vi "Get Field.vi"(0 "Z-Axis Communications Config":T1={"GPIB address"=22, "GPIB bus"=0, "connection ID"=refnum, "IP"="111.111.111.1", "Active Comm Interface"=0, "Serial Port"="", "Programmer Type"=0} {"Active Comm Interface" items=["TCP/IP (Model 430 Only)", "RS232", "IEEE488"]; "Programmer Type" items=["Model 430", "Model 420"]}, 3 "error in":T2) -> (4 "Response":bool, 6 "Field(T)":dbl format="%.3f", 8 "error out":T2)   [LabVIEW 2019]
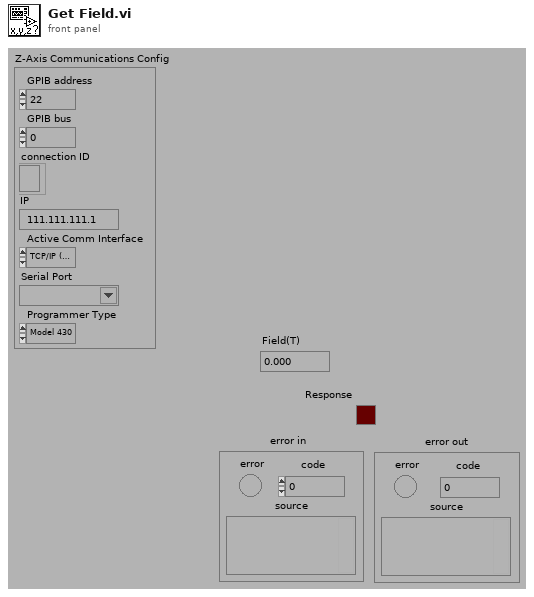
[diagram p1: front panel]
types:
  T1 = cluster{"GPIB address":i16, "GPIB bus":i16, "connection ID":refnum<k5>, "IP":string, "Active Comm Interface":u16, "Serial Port":refnum<visa-resource-name>, "Programmer Type":u16}
  T2 = cluster{"error":bool, "code":i32, "source":string}
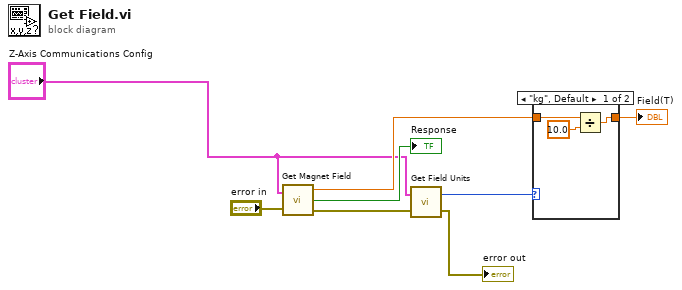
[diagram p0: block diagram]
diagram:
  n1 = call "Get Magnet Field.vi"("Z-Axis Communications Config"="Z-Axis Communications Config", "error in"="error in") -> ("Magnet Field (kG)"=w8:dbl, "Instrument Responded?"=→"Response":bool, "error out"=w5:T2)
  n2 = call "Get Field Units.vi"("error in"=w5, "Z-Axis Communications Config"="Z-Axis Communications Config") -> ("error out"=→"error out":T2, "Field Units"=w4:enum16{"kg", "t"})
  n3 = case shown="\"kg\", Default" w4 {
    tunnel: w8 -> [w10 w12]
    tunnel: [w9 w12] -> w7
    frame "kg", Default {
      n4 = Divide(x=w10, y=10.0) -> (x/y=w9:dbl)
    }
    frame "t" {
    }
  }
  "Field(T)" <- w7
